vi "SwapInstanceVIUnusedName2 55.vi"(6 "Bindata & descr in":T1, 7 "type":u64, 8 "error in (no error)":errorcluster, 9 "dims":u8=3 min=1 max=3, 11 "kwarg_name":string="testarg") -> (0 "error out":errorcluster, 1 "Array 3D":u64[][][](array[numeric]), 2 "Array 2D":u64[][](array[numeric]), 3 "Array 1D":u64[](array[numeric]), 4 "Bindata & descr out":T1, 5 "bindata":u8[](array[numeric]))   [LabVIEW 2018]
uses:
  Bindata&description.ctl
  Bindata description.ctl
  c23e7d99-d8c2-4007-9178-8f398a6e5871.vi
  57e89cd7-ee4c-4905-bb48-2057cad012ca.vi
  e781317f-f964-4505-b238-659dac32b7de.vi
  37b28a3c-a4d4-4f8b-b46c-55d3896ba0c1.vi
  57e89cd7-ee4c-4905-bb48-2057cad012ca.vi/be8b0598-fa53-4c36-a9c1-d947c44d6a07.vi
  e781317f-f964-4505-b238-659dac32b7de.vi/e1ae0052-a496-4b08-832a-36a30338dd18.vi
  37b28a3c-a4d4-4f8b-b46c-55d3896ba0c1.vi/18d02e68-3eb8-4c9c-b7bd-583e8a41748f.vi
  57e89cd7-ee4c-4905-bb48-2057cad012ca.vi/be8b0598-fa53-4c36-a9c1-d947c44d6a07.vi/30770f18-8626-4aec-912e-36b68445d8ad.vi
  e781317f-f964-4505-b238-659dac32b7de.vi/e1ae0052-a496-4b08-832a-36a30338dd18.vi/e5defd6c-cfa3-4191-8490-55ed9c034790.vi
  37b28a3c-a4d4-4f8b-b46c-55d3896ba0c1.vi/18d02e68-3eb8-4c9c-b7bd-583e8a41748f.vi/0f647ace-182c-476e-acea-c35a21798b97.vi
  57e89cd7-ee4c-4905-bb48-2057cad012ca.vi/be8b0598-fa53-4c36-a9c1-d947c44d6a07.vi/30770f18-8626-4aec-912e-36b68445d8ad.vi/f6c70076-b9b9-4a75-aeba-7cce0600d211.vi
  e781317f-f964-4505-b238-659dac32b7de.vi/e1ae0052-a496-4b08-832a-36a30338dd18.vi/e5defd6c-cfa3-4191-8490-55ed9c034790.vi/6ca18de2-3725-46e0-9a4a-1a72c098b4b8.vi
  37b28a3c-a4d4-4f8b-b46c-55d3896ba0c1.vi/18d02e68-3eb8-4c9c-b7bd-583e8a41748f.vi/0f647ace-182c-476e-acea-c35a21798b97.vi/9f698e74-811e-4696-8636-71dea3fbeb4e.vi
  check ID validity.vi
  LV-Julia_ZMQ-Roundtrip_lib.lvlib
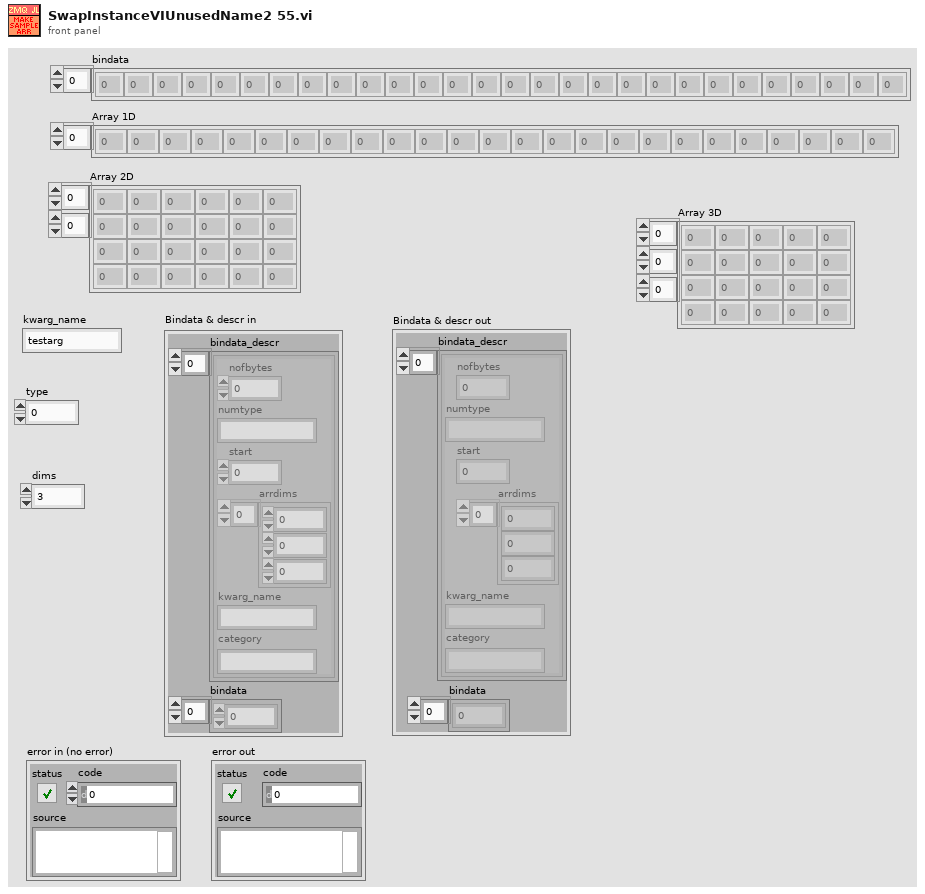
[diagram p1: front panel]
types:
  T1 = typedef "Bindata&description.ctl" = cluster{"bindata_descr":T2[], "bindata":u8[]}
  T2 = typedef "LV-Julia_ZMQ-Roundtrip_lib.lvlib/Bindata description.ctl" = cluster{"nofbytes":i32, "numtype":string, "start":i32, "arrdims":i32[], "kwarg_name":string, "category":string}
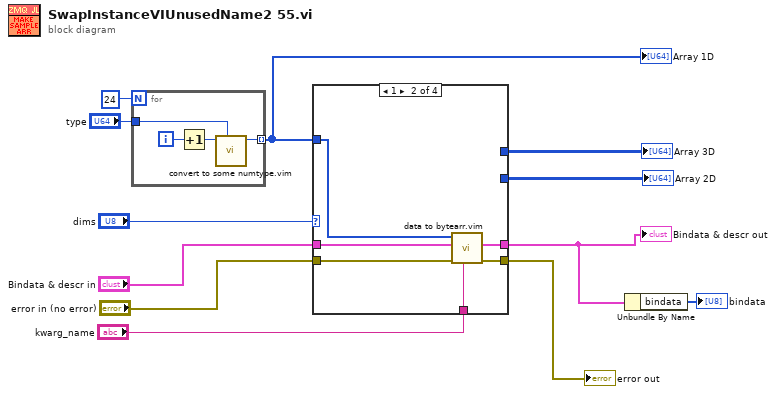
[diagram p0: block diagram]
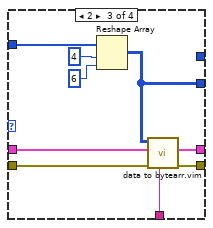
[diagram p3: hidden frame]
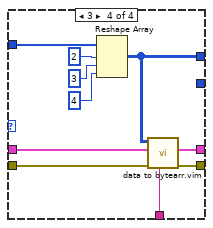
[diagram p4: hidden frame]
diagram:
  n1 = for {
    N: 24 -> [_]
    tunnel: [w14] -> w11 mode=indexing
    tunnel: "type" -> [w13]
    i -> [w16]
    n2 = Increment(x=w16) -> (x+1=w15:i32)
    n3 = call "convert to some numtype.vim"("type"=w13, "Numeric in"=w15) -> ("Numeric out"=w14:u64)  [unwired: 9 in]
  }
  "Array 1D" <- w11
  n4 = case shown="1" "dims" {
    tunnel: [_ _ _ w42] -> w12
    tunnel: w11 -> [_ w23 w30 w38]
    tunnel: "kwarg_name" -> [_ w22 w29 w37]
    tunnel: "error in (no error)" -> [w17 w21 w28 w36]
    tunnel: [w17 w20 w27 w35] -> w5
    tunnel: [_ w19 w26 w34] -> w2
    tunnel: [_ _ w25 _] -> w4
    tunnel: "Bindata & descr in" -> [_ w18 w24 w33]
    frame 0, Default {
    }
    frame 1 {
      n5 = call "data to bytearr.vim"("kwarg_name"=w22, "error in (no error)"=w21, "Bindata & descr in"=w18, "data in"=w23) -> ("error out"=w20:errorcluster, "Bindata & descr out"=w19:T1)  [unwired: 5 in, 1 out]
    }
    frame 2 {
      n6 = Reshape Array(w30, 4 ("dimension size"), 6 ("dimension size")) -> (w25:u64[][])
      n7 = call "data to bytearr.vim"("kwarg_name"=w29, "error in (no error)"=w28, "Bindata & descr in"=w24, "data in"=w25) -> ("error out"=w27:errorcluster, "Bindata & descr out"=w26:T1)  [unwired: 5 in, 1 out]
    }
    frame 3 {
      n8 = Reshape Array(w38, 2 ("dimension size"), 3 ("dimension size"), 4 ("dimension size")) -> (w42:u64[][][])
      n9 = call "data to bytearr.vim"("kwarg_name"=w37, "error in (no error)"=w36, "Bindata & descr in"=w33, "data in"=w42) -> ("error out"=w35:errorcluster, "Bindata & descr out"=w34:T1)  [unwired: 5 in, 1 out]
    }
  }
  "Array 3D" <- w12
  "Bindata & descr out" <- w2
  "error out" <- w5
  "Array 2D" <- w4
  n10 = Unbundle By Name(w2) -> ("bindata"=→"bindata":u8[])
